vi "avg joystick and frame trig lick3.vi"(10 "stop in":refnum<vi>, 11 "Joystick File":path=path "C:/Users/Mackenzie Amoroso/Desktop/junk") -> ()   [LabVIEW 2012]
uses:
  <resource>/objmgr/daqmx.rc
  <vilib>/DAQmx/read.llb/DAQmx Read (Analog 2D DBL NChan NSamp).vi
panel:
  out "frame count 2":u32
  in  "stop 2":bool
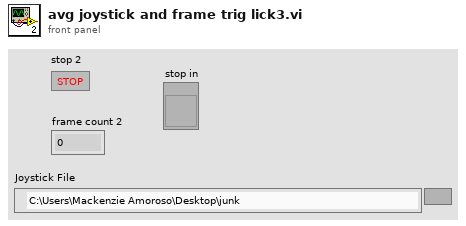
[diagram p1: front panel]
types:
  T1 = enum16{"open", "replace", "create", "open or create", "replace or create", "replace or create with confirmation"}
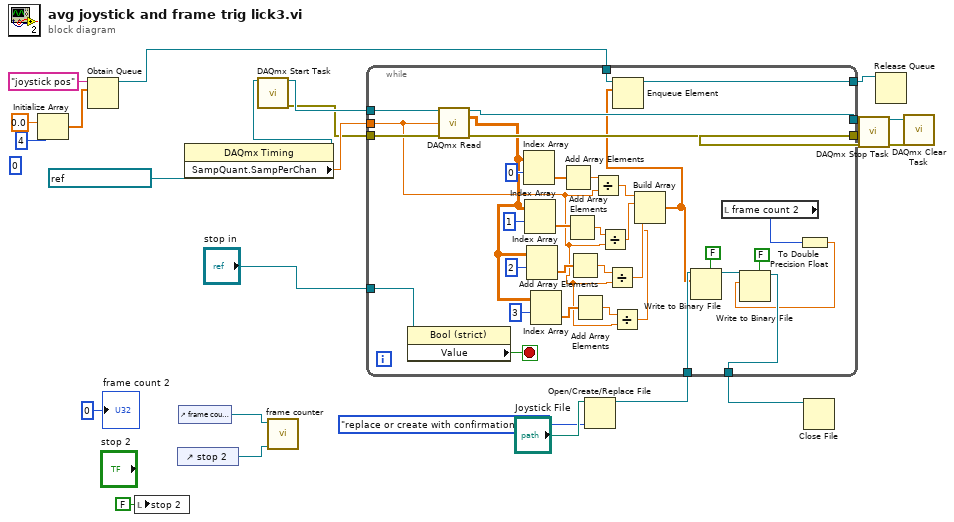
[diagram p0: block diagram]
diagram:
  (unwired) 0 ("dimension size")
  n1 = Initialize Array(0.0 ("element"), 4 ("dimension size")) -> (w12:dbl[])
  n2 = Obtain Queue(name (unnamed)="joystick pos", element data type=w12) -> (queue out=w11:refnum<queue>)  [unwired: 3 in, 2 out]
  n3 = local write "stop 2"(FALSE ("stop")) -> ()
  n4 = control-ref of="stop 2"() -> (w3:refnum<vi>)
  n5 = control-ref of="frame count 2"() -> (w4:refnum<vi>)
  n6 = property class="DAQmx Timing"(reference=refnum<k21> "JOYSTICKLICK" ("task/channels in")) -> (reference out=w20:refnum<k21>, "SampQuant.SampPerChan"=w19:dbl)  [unwired: 1 in, 1 out]
  n7 = call <vilib>:"DAQmx Start Task.vi"("task/channels in"=w20) -> ("task out"=w22:refnum<k21>, "error out"=w18:errorcluster)  [unwired: 13 in]
  n8 = call "frame counter.vi"("stop ref"=w3, "frame count ref"=w4) -> ()  [unwired: 10 in]
  n9 = Open/Create/Replace File(file path (use dialog)="Joystick File", operation (0:open)=T1."replace or create with confirmation") -> (refnum out=w7:refnum<file>)  [unwired: 4 in, 2 out]
  n10 = while {
    tunnel: w22 -> [w58]
    tunnel: w19 -> [w31]
    tunnel: w18 -> [w57]
    tunnel: [w56] -> w17
    tunnel: [w55] -> w16
    tunnel: w11 -> [w47]
    tunnel: [w45] -> w10
    tunnel: w7 -> [w44]
    tunnel: [w27] -> w6
    tunnel: "stop in" -> [w41]
    stop <- w42 stop-if-true
    n11 = property class="Bool (strict)"(reference=w41) -> ("Value"=w42:bool)  [unwired: 1 in, 2 out]
    n12 = call-poly <vilib>:"DAQmx Read.vi"("task/channels in"=w58, "number of samples per channel"=w31, "error in"=w57) -> ("task out"=w56:refnum<k21>, "data"=w35:dbl[][], "error out"=w55:errorcluster)  [unwired: 10 in]
    n13 = Index Array(array=w35, index (row)=0) -> (element=w52:dbl[])  [unwired: 1 in]
    n14 = Index Array(array=w35, index (row)=1) -> (element=w51:dbl[])  [unwired: 1 in]
    n15 = Index Array(array=w35, index (row)=2) -> (element=w39:dbl[])  [unwired: 1 in]
    n16 = Index Array(array=w35, index (row)=3) -> (element=w32:dbl[])  [unwired: 1 in]
    n17 = Add Array Elements(numeric array=w52) -> (sum=w50:dbl)
    n18 = Add Array Elements(numeric array=w51) -> (sum=w49:dbl)
    n19 = Add Array Elements(numeric array=w39) -> (sum=w38:dbl)
    n20 = Add Array Elements(numeric array=w32) -> (sum=w33:dbl)
    n21 = Divide(x=w50, y=w31) -> (x/y=w48:dbl)
    n22 = Divide(x=w49, y=w31) -> (x/y=w46:dbl)
    n23 = Divide(x=w38, y=w31) -> (x/y=w37:dbl)
    n24 = Divide(x=w33, y=w31) -> (x/y=w30:dbl)
    n25 = Build Array(w48, w46, w37, w30) -> (w36:dbl[])
    n26 = Enqueue Element(queue=w47, element=w36) -> (queue out=w45:refnum<queue>)  [unwired: 2 in, 2 out]
    n27 = Write to Binary File(file (use dialog)=w44, data=w36, 5:FALSE ("prepend array or string size? (T)")) -> (refnum out=w28:refnum<file>)  [unwired: 3 in, 2 out]
    n28 = local read "frame count 2"() -> (w26:u32)
    n29 = To Double Precision Float(number=w26) -> (double precision float=w25:dbl)
    n30 = Write to Binary File(file (use dialog)=w28, data=w25, 5:FALSE ("prepend array or string size? (T)")) -> (refnum out=w27:refnum<file>)  [unwired: 3 in, 2 out]
  }
  n31 = Close File(refnum=w6) -> ()  [unwired: 1 in, 2 out]
  n32 = call <vilib>:"DAQmx Stop Task.vi"("task/channels in"=w17, "error in"=w16) -> ("task out"=w24:refnum<k21>, "error out"=w23:errorcluster)  [unwired: 12 in]
  n33 = Release Queue(queue=w10) -> ()  [unwired: 2 in, 3 out]
  n34 = call <vilib>:"DAQmx Clear Task.vi"("task in"=w24, "error in"=w23) -> ()  [unwired: 13 in, 1 out]
  "frame count 2" <- u32 0 ("frame count")
